vi "HW_ni_Pharse Channel Config.vi"(10 "Paravalues[]":string[](array[string]), 11 "ParaNames[]":string[](array[string])) -> (3 "ChanCFG out":T1={"use"=FALSE, "ChanName"="", "ChanAlias"="", "SampleRate"=1000.0, "SlopeA"=1000.0, "InterceptB"=1000.0, "Unit"=""} {"InterceptB" format="%#_13g"; "SlopeA" format="%#_13g"; "SampleRate" format="%#_13g"})   [LabVIEW 2016]
uses:
  HW_ni_Channel Configuration Structure.ctl
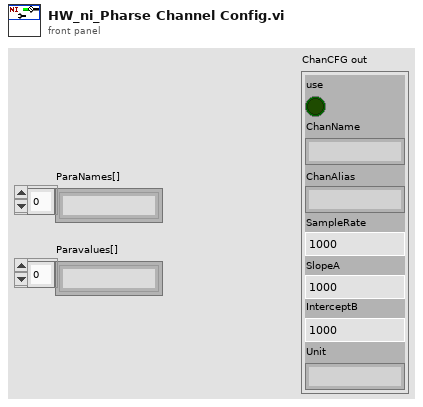
[diagram p1: front panel]
types:
  T1 = typedef "HW_ni_Channel Configuration Structure.ctl" = cluster{"use":bool, "ChanName":string, "ChanAlias":string, "SampleRate":dbl, "SlopeA":dbl, "InterceptB":dbl, "Unit":string}
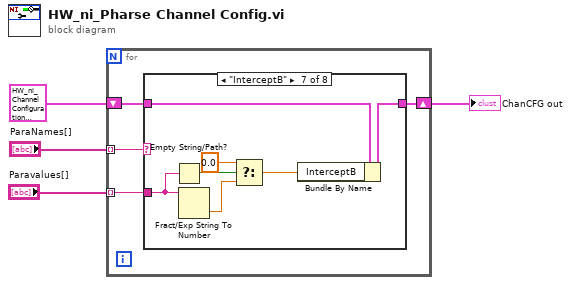
[diagram p0: block diagram]
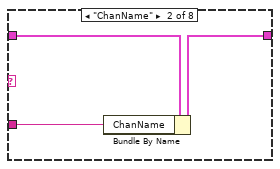
[diagram p3: hidden frame]
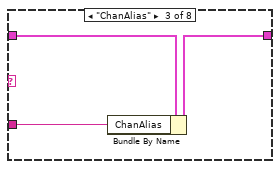
[diagram p4: hidden frame]
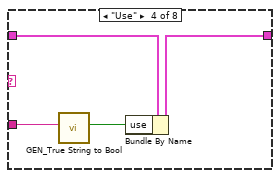
[diagram p5: hidden frame]
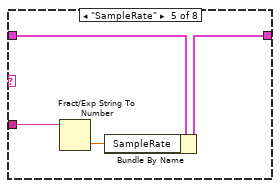
[diagram p6: hidden frame]
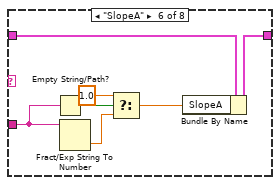
[diagram p7: hidden frame]
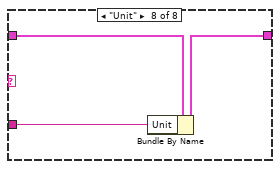
[diagram p8: hidden frame]
diagram:
  n1 = for {
    shift-right: [w5] -> w1
    shift-left: T1 {"use"=FALSE, "ChanName"="", "ChanAlias"="", "SampleRate"=1000.0, "SlopeA"=1000.0, "InterceptB"=1000.0, "Unit"=""} ("ChanCFG out") -> [w8]
    tunnel: "ParaNames[]" -> [w7] mode=indexing
    tunnel: "Paravalues[]" -> [w6] mode=indexing
    n2 = case shown="\"InterceptB\"" w7 {
      tunnel: w8 -> [w9 w12 w15 w19 w23 w30 w37 w40]
      tunnel: w6 -> [_ w11 w14 w18 w21 w28 w35 w38]
      tunnel: [w9 w10 w13 w17 w22 w29 w36 w39] -> w5
      frame Default {
      }
      frame "ChanName" {
        n3 = Bundle By Name(cluster=w12, "ChanName"=w11) -> (w10:T1)
      }
      frame "ChanAlias" {
        n4 = Bundle By Name(cluster=w15, "ChanAlias"=w14) -> (w13:T1)
      }
      frame "Use" {
        n5 = call "GEN_True String to Bool.vi"("string in"=w18) -> ("true?"=w16:bool)  [unwired: 10 in]
        n6 = Bundle By Name(cluster=w19, "use"=w16) -> (w17:T1)
      }
      frame "SampleRate" {
        n7 = Fract/Exp String To Number(string=w21) -> (number=w20:dbl)  [unwired: 3 in, 1 out]
        n8 = Bundle By Name(cluster=w23, "SampleRate"=w20) -> (w22:T1)
      }
      frame "SlopeA" {
        n9 = Empty String/Path?(string/path=w28) -> (empty?=w27:bool)
        n10 = Fract/Exp String To Number(string=w28) -> (number=w25:dbl)  [unwired: 3 in, 1 out]
        n11 = Select(t=1.0, s=w27, f=w25) -> (s? t:f=w24:dbl)
        n12 = Bundle By Name(cluster=w30, "SlopeA"=w24) -> (w29:T1)
      }
      frame "InterceptB" {
        n13 = Empty String/Path?(string/path=w35) -> (empty?=w34:bool)
        n14 = Fract/Exp String To Number(string=w35) -> (number=w32:dbl)  [unwired: 3 in, 1 out]
        n15 = Select(t=0.0, s=w34, f=w32) -> (s? t:f=w31:dbl)
        n16 = Bundle By Name(cluster=w37, "InterceptB"=w31) -> (w36:T1)
      }
      frame "Unit" {
        n17 = Bundle By Name(cluster=w40, "Unit"=w38) -> (w39:T1)
      }
    }
  }
  "ChanCFG out" <- w1
